vi "encodeStream.vi"(8 "error in (no error)":errorcluster, 11 "tBSONTimestamp in":refnum<class "tBSONTimestamp.lvclass">) -> (0 "error out":errorcluster, 2 "Byte Array":u8[](array[numeric]), 3 "tBSONTimestamp out":refnum<class "tBSONTimestamp.lvclass">)   [LabVIEW 2013, in "BSON.lvlib" / "tBSONTimestamp.lvclass"]
uses:
  tBSONTimestamp.lvclass
  tBSONElement/tBSONElement.lvclass
  getValue.vi
  BSON.lvlib
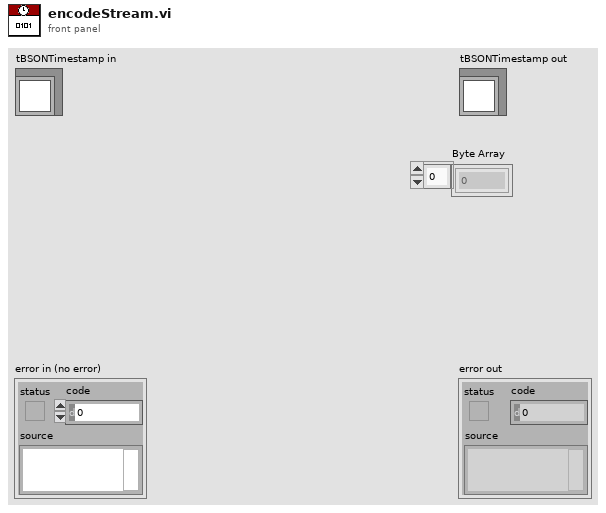
[diagram p1: front panel]
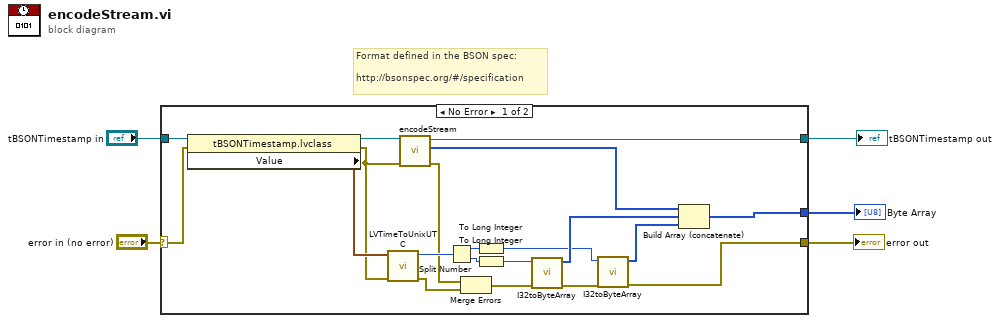
[diagram p0: block diagram]
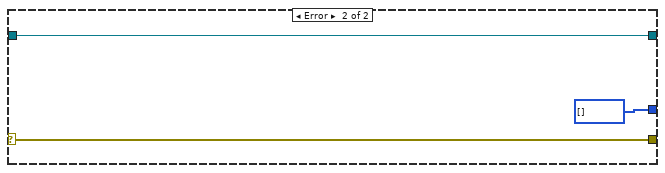
[diagram p2: hidden frame]
diagram:
  # "Format defined in the BSON spec:\n\nhttp://bsonspec.org/#/specification"
  n1 = case shown="No Error" "error in (no error)" {
    selector: "error in (no error)" -> [w24 w27]
    tunnel: "tBSONTimestamp in" -> [w25 w28]
    tunnel: [w6 w28] -> w1
    tunnel: [w15 w27] -> w3
    tunnel: [w23 u8[] []] -> w2
    frame No Error {
      n2 = property class="tBSONTimestamp.lvclass"(reference=w25, error in=w24) -> (reference out=w10:refnum<class "tBSONTimestamp.lvclass">, error out=w9:errorcluster, "Value"=w21:timestamp)
      n3 = call "LVTimeToUnixUTC.vi"("error in"=w9, "Local Time Stamp"=w21) -> ("error out"=w22:errorcluster, "Unix Time (in milliseconds)"=w20:u64)  [unwired: 8 in]
      n4 = call-parent "encodeStream.vi"("error in (no error)"=w9, "tBSONElement in"=w10) -> ("error out"=w8:errorcluster, "Byte Array"=w7:u8[], "tBSONElement out"=w6:refnum<class "tBSONTimestamp.lvclass">)  [unwired: 7 in]
      n5 = Split Number(x=w20) -> (hi(x)=w14:u32, lo(x)=w13:u32)
      n6 = Merge Errors(w8, w22) -> (w19:errorcluster)
      n7 = To Long Integer(number=w14) -> (32bit integer=w12:i32)
      n8 = To Long Integer(number=w13) -> (32bit integer=w11:i32)
      n9 = call "I32toByteArray.vi"("error in (no error)"=w19, "I32"=w11) -> ("error out"=w17:errorcluster, "LittleEndianByteArray"=w18:u8[])  [unwired: 8 in]
      n10 = call "I32toByteArray.vi"("error in (no error)"=w17, "I32"=w12) -> ("error out"=w15:errorcluster, "LittleEndianByteArray"=w16:u8[])  [unwired: 8 in]
      n11 = Build Array (concatenate)(w7, w18, w16) -> (w23:u8[])
    }
    frame Error {
    }
  }
  "error out" <- w3
  "tBSONTimestamp out" <- w1
  "Byte Array" <- w2
